vi "Destroy User Events.vi"(8 "error in (no error)":errorcluster, 11 "User Events":T1) -> (0 "error out":errorcluster)   [LabVIEW 2014, in "User Events.lvlib"]
doc: "Destroy the user event, even if there is an incoming error."
uses:
  User Events.lvlib
  User Events.ctl
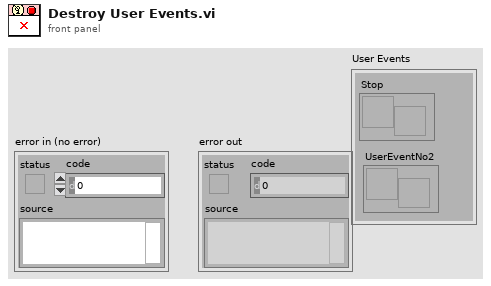
[diagram p1: front panel]
types:
  T1 = typedef "User Events.lvlib/User Events.ctl" = cluster{"Stop":refnum<user-event>, "UserEventNo2":refnum<user-event>}
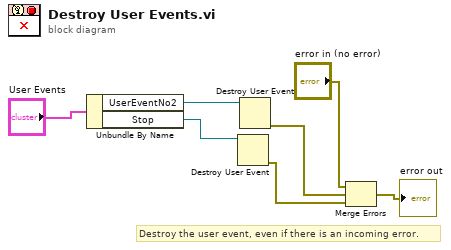
[diagram p0: block diagram]
diagram:
  # "Destroy the user event, even if there is an incoming error."
  n1 = Unbundle By Name("User Events") -> ("UserEventNo2"=w3:refnum<user-event>, "Stop"=w4:refnum<user-event>)
  n2 = Destroy User Event(user event=w4) -> (error out=w7:errorcluster)  [unwired: 1 in]
  n3 = Destroy User Event(user event=w3) -> (error out=w2:errorcluster)  [unwired: 1 in]
  n4 = Merge Errors("error in (no error)", w2, w7) -> (→"error out":errorcluster)
